vi "xml.numeric.vi"(10 "Value":variant, 11 "MsgSerializer.XML in":refnum<class "MsgSerializer.XML.lvclass">) -> (3 "string":string)   [LabVIEW 2013, in "Caraya.lvlib" / "MsgSerializer.XML.lvclass"]
uses:
  MsgSerializer.XML.lvclass
  MsgSerializer.XML.lvclass/MsgSerializer.XML.ctl
  MsgSerializer/MsgSerializer.lvclass/MsgSerializer.ctl
  MsgSerializer/MsgSerializer.lvclass
  <vilib>/Utility/VariantDataType/VariantType.lvlib
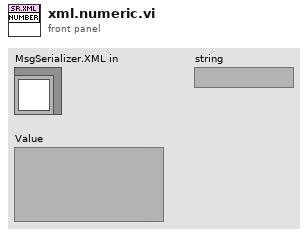
[diagram p1: front panel]
types:
  T1 = typedef "VariantType.lvlib/Type.ctl" = enum8{"Invalid Type", "Void", "I8", "I16", "I32", "I64", "U8", "U16", "U32", "U64", "Single Float", "Double Float", "Extended Float", "Single Complex", "Double Complex", "Extended Complex", "Enum U8", "Enum U16", "Enum U32", "Enum U64", "Single Float With Unit", "Double Float With Unit", "Extended Float With Unit", "Single Complex with Unit", "Double Complex with Unit", "Extended Complex with Unit", "Boolean", "String", "Path", "Picture", "Tag", "Array", "Cluster", "Variant", "LV Variant", "Waveform", "Timestamp", "Digital Waveform", "Digital Data", "ExpressData", "Refnum", "External Data", "VI", "Poly VI", "LabVIEW Class Instance", "Fixed Point"}
  T2 = typedef "Caraya.lvlib/MsgSerializer.XML.lvclass/format -- enum.ctl" = enum16{"value", "tag", "property"}
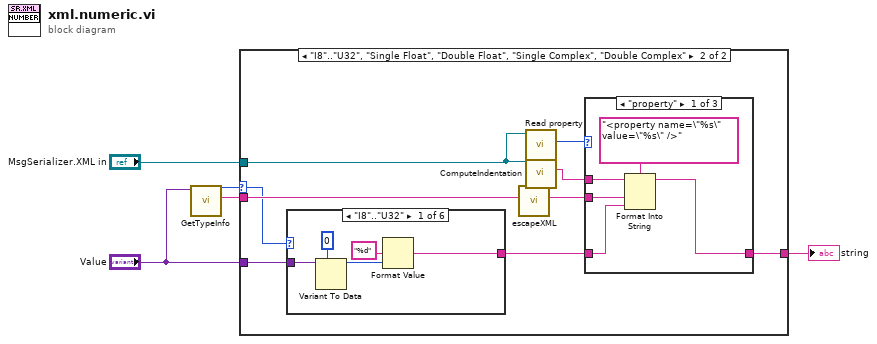
[diagram p0: block diagram]
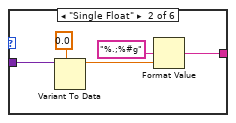
[diagram p3: hidden frame]
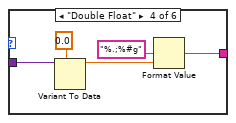
[diagram p5: hidden frame]
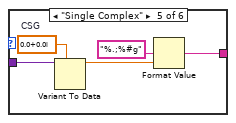
[diagram p6: hidden frame]
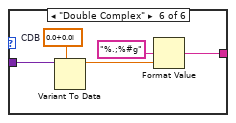
[diagram p7: hidden frame]
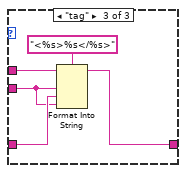
[diagram p9: hidden frame]
diagram:
  n1 = call <vilib>:"GetTypeInfo.vi"("Variant"="Value") -> ("Name"=w4:string, "Type Enum"=w1:T1)  [unwired: 6 in, 3 out]
  n2 = case shown="\"I8\"..\"U32\", \"Single Float\", \"Double Float\", \"Single Complex\", \"Double Complex\"" w1 {
    selector: w1 -> [_ w6]
    tunnel: "Value" -> [_ w13]
    tunnel: w4 -> [_ w11]
    tunnel: "MsgSerializer.XML in" -> [_ w9]
    tunnel: [_ w8] -> w2
    frame Default {
    }
    frame "I8".."U32", "Single Float", "Double Float", "Single Complex", "Double Complex" {
      n3 = case shown="\"I8\"..\"U32\"" w6 {
        tunnel: w13 -> [w19 w21 _ w26 w32 w37]
        tunnel: [w18 w20 _ w25 w31 w36] -> w7
        frame "I8".."U32" {
          n4 = Variant To Data(type=i64 0, Variant=w19) -> (data=w15:i64)  [unwired: 1 in, 1 out]
          n5 = Format Value(format string="%d", value (0)=w15) -> (output string=w18:string)  [unwired: 1 in]
        }
        frame "Single Float" {
          n6 = Variant To Data(type=sgl 0.0, Variant=w21) -> (data=w24:sgl)  [unwired: 1 in, 1 out]
          n7 = Format Value(format string="%.;%#g", value (0)=w24) -> (output string=w20:string)  [unwired: 1 in]
        }
        frame Default {
        }
        frame "Double Float" {
          n8 = Variant To Data(type=0.0, Variant=w26) -> (data=w29:dbl)  [unwired: 1 in, 1 out]
          n9 = Format Value(format string="%.;%#g", value (0)=w29) -> (output string=w25:string)  [unwired: 1 in]
        }
        frame "Single Complex" {
          w30 = csg 0.0+0.0i  # CSG
          n10 = Variant To Data(type=w30, Variant=w32) -> (data=w34:csg)  [unwired: 1 in, 1 out]
          n11 = Format Value(format string="%.;%#g", value (0)=w34) -> (output string=w31:string)  [unwired: 1 in]
        }
        frame "Double Complex" {
          w35 = cdb 0.0+0.0i  # CDB
          n12 = Variant To Data(type=w35, Variant=w37) -> (data=w39:cdb)  [unwired: 1 in, 1 out]
          n13 = Format Value(format string="%.;%#g", value (0)=w39) -> (output string=w36:string)  [unwired: 1 in]
        }
      }
      n14 = call "escapeXML.vi"("Input String"=w11) -> ("XML-escaped String"=w12:string)  [unwired: 10 in]
      n15 = call "Read property.vi"("MsgSerializer.XMLProperty in"=w9) -> ("format"=w14:T2)  [unwired: 9 in, 1 out]
      n16 = call "ComputeIndentation.vi"("MsgSerializer in"=w9) -> ("indentation"=w10:string)  [unwired: 10 in]
      n17 = case shown="\"property\"" w14 {
        tunnel: w7 -> [w43 w45 w49]
        tunnel: [w42 w45 w46] -> w8
        tunnel: w10 -> [w40 _ w48]
        tunnel: w12 -> [w41 _ w47]
        frame "property" {
          n18 = Format Into String(format string="<property name=\"%s\" value=\"%s\" />" ("name"), initial string=w40, w41, w43) -> (resulting string=w42:string)  [unwired: 1 in, 1 out]
        }
        frame "value" {
        }
        frame "tag" {
          n19 = Format Into String(format string="<%s>%s</%s>" ("name"), initial string=w48, w47, w49, w47) -> (resulting string=w46:string)  [unwired: 1 in, 1 out]
        }
      }
    }
  }
  "string" <- w2
